vi "Read Voltage.vi"(8 "error in (no error)":errorcluster, 11 "34972A in":refnum<class "34972A.lvclass">) -> (0 "error out":errorcluster, 2 "Voltage":dbl, 3 "34972A out":refnum<class "34972A.lvclass">)   [LabVIEW 2020, in "34972A.lvclass"]
uses:
  34972A.lvclass
  34972A.lvclass/34972A.ctl
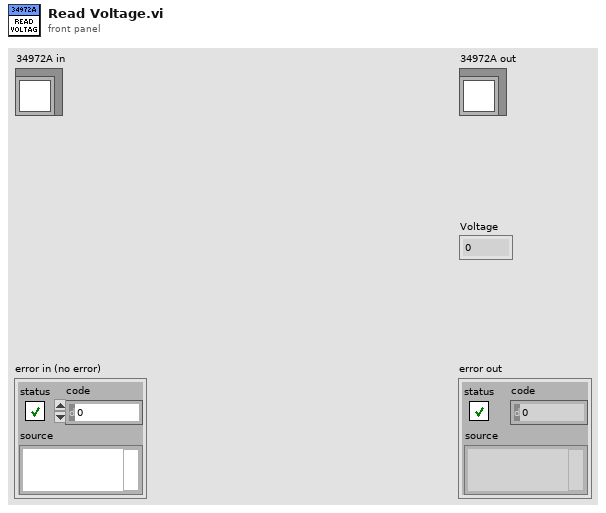
[diagram p1: front panel]
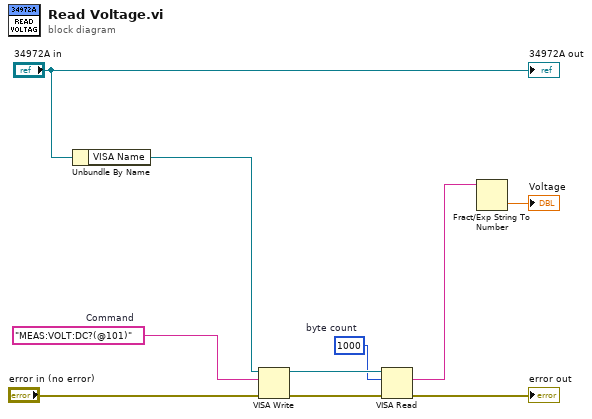
[diagram p0: block diagram]
diagram:
  w3 = u32 1000  # byte count
  w9 = "MEAS:VOLT:DC?(@101)"  # Command
  n1 = Unbundle By Name("34972A in") -> ("VISA Name"=w8:refnum<visa-resource-name>)
  n2 = VISA Write(VISA resource name=w8, write buffer=w9, error in (no error)="error in (no error)") -> (VISA resource name out=w4:refnum<visa-resource-name>, error out=w6:errorcluster)  [unwired: 1 out]
  n3 = VISA Read(VISA resource name=w4, byte count=w3, error in (no error)=w6) -> (read buffer=w1:string, error out=→"error out":errorcluster)  [unwired: 2 out]
  n4 = Fract/Exp String To Number(string=w1) -> (number=→"Voltage":dbl)  [unwired: 3 in, 1 out]
  "34972A out" <- "34972A in"
